vi "CAN Get Status.vi"(8 "error in (no error)":errorcluster, 11 "Channel":u16) -> (0 "error out":errorcluster, 2 "Channel out":u16, 3 "function return":u32)   [LabVIEW 2025, in "PCAN2023.lvlib"]
doc: "Gets the current status of a PCAN Channel\n\n\nTPCANStatus __stdcall CAN_GetStatus(\n TPCANHandle Channel);"
uses:
  PCAN2023.lvlib
  x64/PCANBasic.dll
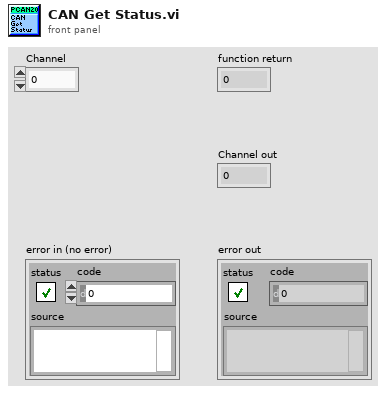
[diagram p1: front panel]
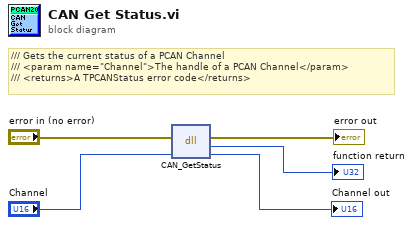
[diagram p0: block diagram]
diagram:
  # "/// Gets the current status of a PCAN Channel\n/// <param name=\"Channel\">The handle of a PCAN Channel</param>\n/// <returns>A TPCANStatus error code</returns>"
  n1 = dll-call lib="C:/UTP/LabView/Communication Handle/PCAN2023/x64/PCANBasic.dll" fn="CAN_GetStatus"(error in="error in (no error)", "Channel"="Channel") -> (error out=→"error out":errorcluster, "return type"=→"function return":u32, "Channel"=→"Channel out":u16)  [unwired: 2 in, 1 out]
